vi "Paths.vi"() -> (2 "Icon Path":path, 3 "UDL Path":path)   [LabVIEW 2020]
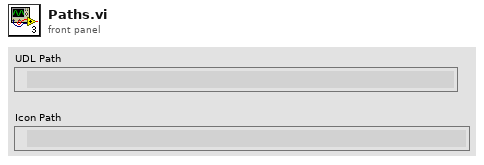
[diagram p1: front panel]
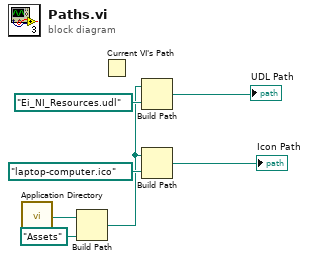
[diagram p0: block diagram]
diagram:
  n1 = call <vilib>:"Application Directory.vi"() -> ("Application Directory"=w2:path)
  n2 = Build Path(base path=w2, name or relative path=path "Assets") -> (appended path=w1:path)
  n3 = Current VI's Path() -> ()  [unwired: 1 out]
  n4 = Build Path(base path=w1, name or relative path=path "Ei_NI_Resources.udl") -> (appended path=→"UDL Path":path)
  n5 = Build Path(base path=w1, name or relative path=path "laptop-computer.ico") -> (appended path=→"Icon Path":path)
